vi "getLatestDAQmxTimestamp.vi"() -> (2 "DAQmx timestamp available?":bool, 3 "Timestamp":timestamp)   [LabVIEW 2017]
uses:
  Latest DAQmx timestamp.vi
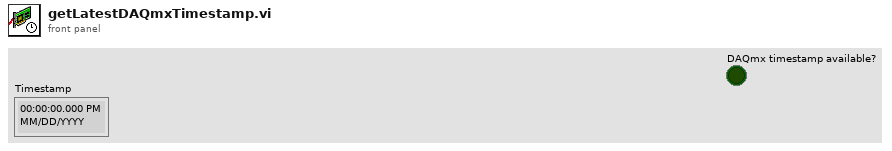
[diagram p1: front panel]
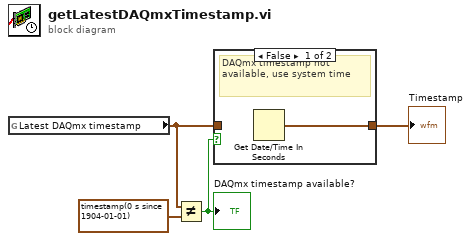
[diagram p0: block diagram]
diagram:
  n1 = global read "Latest DAQmx timestamp.vi" "Latest DAQmx timestamp"() -> (w4:timestamp)
  n2 = Not Equal?(x=w4, y=timestamp(0 s since 1904-01-01) ("Latest DAQmx timestamp")) -> (x != y?=w3:bool)
  "DAQmx timestamp available?" <- w3
  n3 = case shown="False" w3 {
    tunnel: [w5 w6] -> w1
    tunnel: w4 -> [_ w6]
    frame False {
      # "DAQmx timestamp not available, use system time"
      n4 = Get Date/Time In Seconds() -> (seconds since 1Jan1904=w5:timestamp)
    }
    frame True {
      # "Use DAQmx latest timestamp"
    }
  }
  "Timestamp" <- w1
